vi "sub_UI_data_clear.vi"   [LabVIEW 2016]
uses:
  ctl/UI_cmd-ctl.ctl
  ctl/Data_buf_cmd.ctl
types:
  T1 = typedef "UI_cmd-ctl.ctl" = enum16{"default", "create", "read"}
  T2 = typedef "UI_ctl.ctl" = cluster{"Heater temp":refnum<vi>, "Heater chart":refnum<vi>, "vacuum (kpa)":refnum<vi>, "Balance xy graph":refnum<vi>, "Strain chart w cal":refnum<vi>, "Pickup force":refnum<vi>, "Pickup time":refnum<vi>, "Force chart":refnum<vi>, "Force graph T":refnum<vi>, "vacuum chart":refnum<vi>, "vacuum rt":refnum<vi>, "Strain raw graph":refnum<vi>, "Strain raw chart":refnum<vi>, "Bonding time":refnum<vi>, "Bonding force":refnum<vi>, "Balance":refnum<vi>, "Filtered force graph":refnum<vi>, "ROI intensity":refnum<vi>, "Heater_rt":refnum<vi>, "Detach force":refnum<vi>, "Force rt":refnum<vi>, "Mixed signal":refnum<vi>}
  T3 = typedef "Data_buf_cmd.ctl" = enum16{"insert", "default", "create", "clear"}
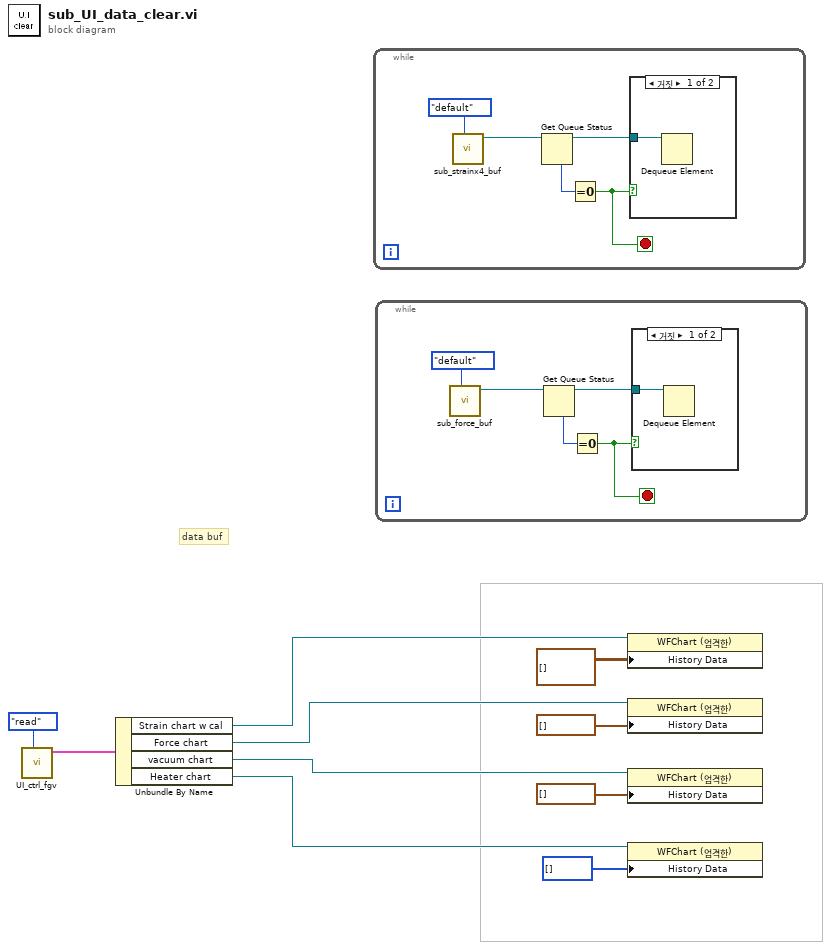
[diagram p0: block diagram]
diagram:
  # "data buf"
  n1 = call "UI_ctrl_fgv.vi"("cmd"=UI_cmd-ctl."read") -> ("UI cluster out"=w9:T2)  [unwired: 10 in]
  n2 = Unbundle By Name(w9) -> ("Strain chart w cal"=w8:refnum<vi>, "Force chart"=w7:refnum<vi>, "vacuum chart"=w6:refnum<vi>, "Heater chart"=w5:refnum<vi>)
  n3 = while {
    stop <- w13 stop-if-true
    n4 = call "sub_strainx4_buf.vi"("cmd"=Data_buf_cmd."default") -> ("queue out"=w11:refnum<queue>)  [unwired: 9 in, 1 out]
    n5 = Get Queue Status(queue=w11) -> (queue out=w14:refnum<queue>, # elements in queue=w15:i32)  [unwired: 2 in, 6 out]
    n6 = Equal To 0?(x=w15) -> (x = 0?=w13:bool)
    n7 = case shown="거짓" w13 {
      tunnel: w14 -> [w16 _]
      frame False {
        n8 = Dequeue Element(queue=w16) -> ()  [unwired: 2 in, 4 out]
      }
      frame True {
      }
    }
  }
  n9 = while {
    stop <- w17 stop-if-true
    n10 = call "sub_force_buf.vi"("cmd"=Data_buf_cmd."default") -> ("queue out"=w20:refnum<queue>)  [unwired: 9 in, 1 out]
    n11 = Get Queue Status(queue=w20) -> (queue out=w18:refnum<queue>, # elements in queue=w19:i32)  [unwired: 2 in, 6 out]
    n12 = Equal To 0?(x=w19) -> (x = 0?=w17:bool)
    n13 = case shown="거짓" w17 {
      tunnel: w18 -> [w22 _]
      frame False {
        n14 = Dequeue Element(queue=w22) -> ()  [unwired: 2 in, 4 out]
      }
      frame True {
      }
    }
  }
  n15 = property class="WFChart (엄격한)"(reference=w8, "History Data"=waveform(dbl)[][] [] ("히스토리 데이터")) -> ()  [unwired: 1 in, 2 out]
  n16 = property class="WFChart (엄격한)"(reference=w7, "History Data"=waveform(dbl)[] [] ("히스토리 데이터")) -> ()  [unwired: 1 in, 2 out]
  n17 = property class="WFChart (엄격한)"(reference=w6, "History Data"=waveform(dbl)[] [] ("히스토리 데이터")) -> ()  [unwired: 1 in, 2 out]
  n18 = property class="WFChart (엄격한)"(reference=w5, "History Data"=i32[] [] ("히스토리 데이터")) -> ()  [unwired: 1 in, 2 out]
